vi "id参数转换.vi"(11 "id":u16) -> (3 "table输出":string)   [LabVIEW 2016, in "斯坦道总氮.lvlib"]
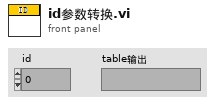
[diagram p1: front panel]
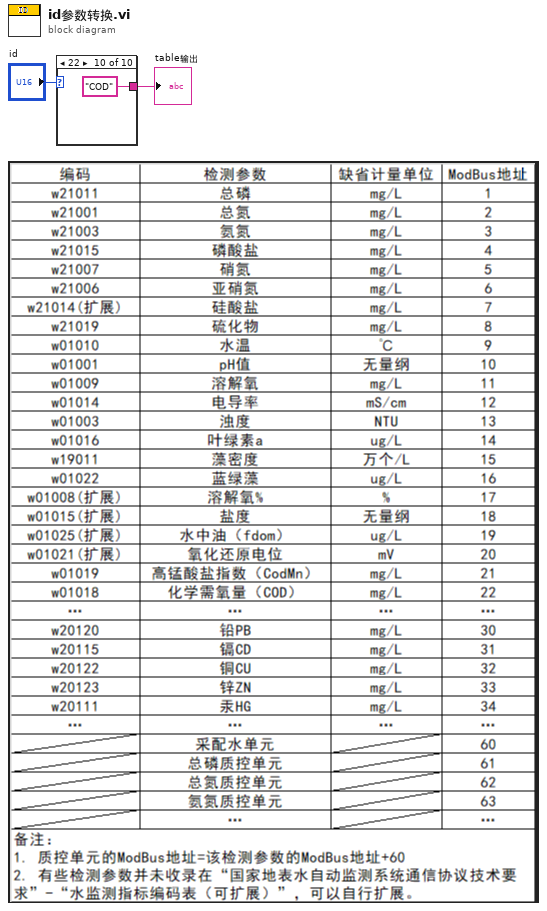
[diagram p0: block diagram]
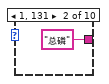
[diagram p3: hidden frame]
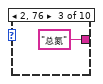
[diagram p4: hidden frame]
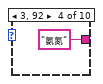
[diagram p5: hidden frame]
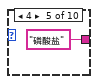
[diagram p6: hidden frame]
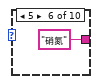
[diagram p7: hidden frame]
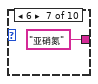
[diagram p8: hidden frame]
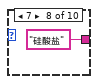
[diagram p9: hidden frame]
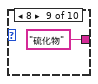
[diagram p10: hidden frame]
diagram:
  n1 = case shown="22" "id" {
    tunnel: [_ "总磷" ("table输入") "总氮" ("table输入") "氨氮" ("table输入") "磷酸盐" ("table输入") "硝氮" ("table输入") "亚硝氮" ("table输入") "硅酸盐" ("table输入") "硫化物" ("table输入") "COD" ("table输入")] -> w2
    frame 0, Default {
    }
    frame 1, 131 {
    }
    frame 2, 76 {
    }
    frame 3, 92 {
    }
    frame 4 {
    }
    frame 5 {
    }
    frame 6 {
    }
    frame 7 {
    }
    frame 8 {
    }
    frame 22 {
    }
  }
  "table输出" <- w2
